vi "Create new PID Loop.vi"(7 "ID":string, 8 "error in (no error)":errorcluster, 9 "output range":T2 {"output low" format="%.2f"; "output high" format="%.2f"}, 10 "PID gains":T3 {"proportional gain (Kc)" format="%.2f"; "integral time (Ti, min)" format="%.2f"}, 11 "PID Parameters":T1) -> (0 "error out":errorcluster, 3 "PID Loop out":refnum<class "PID Loop.lvclass">)   [LabVIEW 2015, in "PID Loop.lvclass"]
uses:
  PID Loop.lvclass
  PID Gains.ctl
  PID Range.ctl
  PID Parameters.ctl
  PID Loop.lvclass/PID Loop.ctl
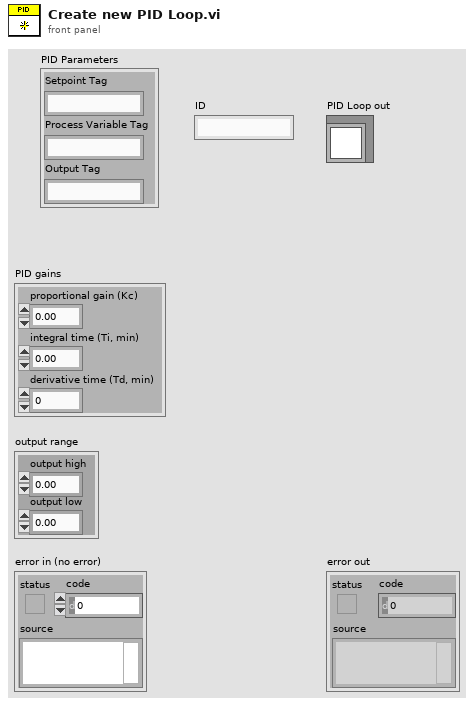
[diagram p1: front panel]
types:
  T1 = typedef "PID Loop.lvclass/PID Parameters.ctl" = cluster{"Setpoint Tag":string, "Process Variable Tag":string, "Output Tag":string}
  T2 = typedef "PID Loop.lvclass/PID Range.ctl" = cluster{"output high":dbl, "output low":dbl}
  T3 = typedef "PID Loop.lvclass/PID Gains.ctl" = cluster{"proportional gain (Kc)":dbl, "integral time (Ti, min)":dbl, "derivative time (Td, min)":dbl}
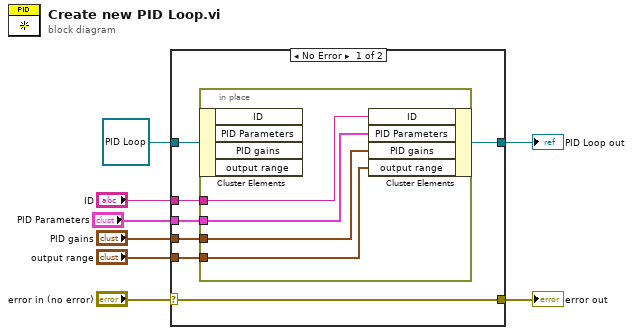
[diagram p0: block diagram]
diagram:
  n1 = case shown="No Error" "error in (no error)" {
    selector: "error in (no error)" -> [w15 w21]
    tunnel: [w15 w21] -> w7
    tunnel: refnum<class "PID Loop.lvclass"> refnum ("PID Loop.lvclass") -> [w14 w20]
    tunnel: "ID" -> [w13 _]
    tunnel: "PID gains" -> [w12 _]
    tunnel: "output range" -> [w11 _]
    tunnel: [w10 w20] -> w2
    tunnel: "PID Parameters" -> [w9 _]
    frame No Error {
      n2 = in-place {
        in-place-border: w13 -> [w19]
        in-place-border: w12 -> [w18]
        in-place-border: w11 -> [w17]
        in-place-border: w9 -> [w16]
        n3 = in-place-cluster #1(w14) -> ()  [unwired: 4 out]
        n4 = in-place-cluster #1("ID"=w19, "PID Parameters"=w16, "PID gains"=w18, "output range"=w17) -> (w10:refnum<class "PID Loop.lvclass">)
      }
    }
    frame Error {
    }
  }
  "error out" <- w7
  "PID Loop out" <- w2
